vi "GetNumberOfIndexes.vi"(0 "reference in":refnum<class "RefferenceA.lvclass">, 11 "Error In":errorcluster) -> (4 "reference out":refnum<class "RefferenceA.lvclass">, 15 "Error Out":errorcluster)   [LabVIEW 2018, in "RefferenceA.lvclass"]
uses:
  RefferenceA.lvclass
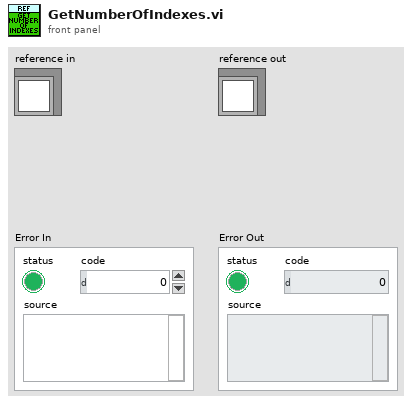
[diagram p1: front panel]
types:
  T1 = typedef "RefferenceA.lvclass/ObjectAttributes.ctl" = cluster{"Attribute1":dbl}
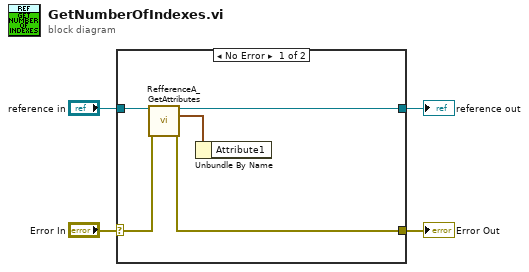
[diagram p0: block diagram]
diagram:
  n1 = case shown="No Error" "Error In" {
    selector: "Error In" -> [w9 w11]
    tunnel: [w7 w11] -> w3
    tunnel: [w5 w10] -> w1
    tunnel: "reference in" -> [w6 w10]
    frame No Error {
      n2 = call "RefferenceA_GetAttributes.vi"("reference in"=w6, "error in (no error)"=w9) -> ("reference out"=w5:refnum<class "RefferenceA.lvclass">, "Data"=w8:T1, "error out"=w7:errorcluster)  [unwired: 10 in, 1 out]
      n3 = Unbundle By Name(w8) -> ()  [unwired: 1 out]
    }
    frame Error {
    }
  }
  "Error Out" <- w3
  "reference out" <- w1
